vi "FPGA Close Reference.vi"(7 "Reset?":T1, 8 "error in (no error)":errorcluster, 11 "FPGA Session In":refnum<class "FPGA Interface Base.lvclass">) -> (0 "error out":errorcluster)   [LabVIEW 2010, in "FPGA Interface Base.lvclass"]
uses:
  <userlib>/_FPGA Interface Advanced Tools/FPGA Interface Base/FPGA Interface Base.lvclass
  <userlib>/_FPGA Interface Advanced Tools/FPGA Interface Wrapper/TypeDefs/Close Attribute.ctl
  <userlib>/_FPGA Interface Advanced Tools/FPGA Interface Base/FPGA Interface Base.lvclass/FPGA Interface Base.ctl
  <vilib>/Utility/error.llb/Error Cluster From Error Code.vi
  <userlib>/_FPGA Interface Advanced Tools/FPGA Interface Wrapper/FPGA Interface Wrapper.lvlib
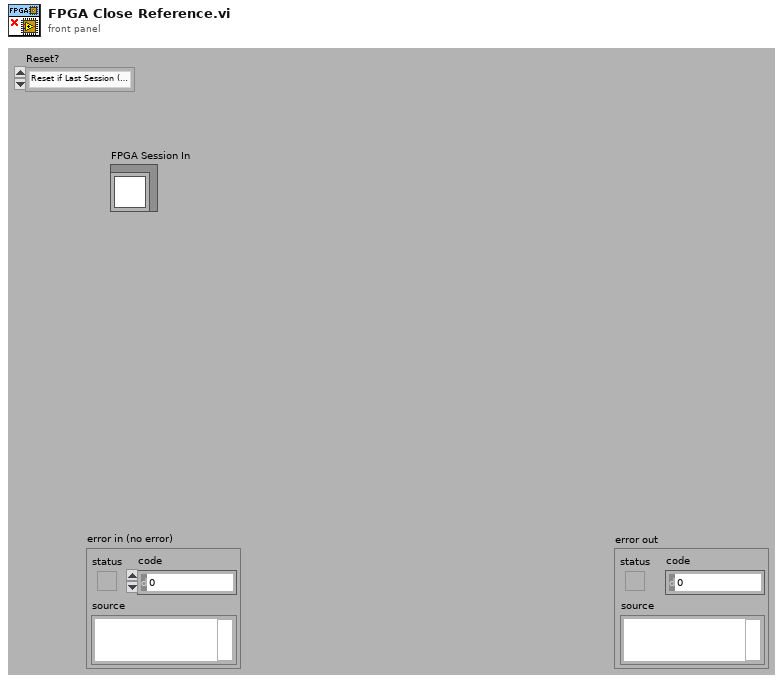
[diagram p1: front panel]
types:
  T1 = typedef "FPGA Interface Wrapper.lvlib/Close Attribute.ctl" = enum32{"Reset if Last Session (Default)", "No Reset"}
  T2 = typedef "FPGA Interface Base.lvclass/FPGA Session.ctl" = refnum<data-value>
  T3 = typedef "FPGA Interface Base.lvclass/FPGA Session Data.ctl" = cluster{"Session Out":u32, "Indicator Scalars":T4, "Indicator Arrays":T6, "Control Scalars":T4, "Control Arrays":T6, "TargetToHost FIFO Channels":T8, "HostToTarget FIFO Channels":T8, "All FIFOs":T9[], "IRQ Context Queue":refnum<queue>}
  T4 = typedef "FPGA Bitfile Utility.lvlib/Scalar Register Set.ctl" = cluster{"Boolean":T5[], "I8":T5[], "I16":T5[], "I32":T5[], "I64":T5[], "U8":T5[], "U16":T5[], "U32":T5[], "U64":T5[]}
  T5 = typedef "FPGA Bitfile Utility.lvlib/Scalar Register.ctl" = cluster{"Address":u32, "Name":string}
  T6 = typedef "FPGA Bitfile Utility.lvlib/Array Register Set.ctl" = cluster{"Boolean":T7[], "I8":T7[], "I16":T7[], "I32":T7[], "I64":T7[], "U8":T7[], "U16":T7[], "U32":T7[], "U64":T7[]}
  T7 = typedef "FPGA Bitfile Utility.lvlib/Array Register.ctl" = cluster{"Address":u32, "Num Elements":u32, "Name":string}
  T8 = typedef "FPGA Bitfile Utility.lvlib/FIFO Channel Set.ctl" = cluster{"Boolean":T9[], "I8":T9[], "I16":T9[], "I32":T9[], "I64":T9[], "U8":T9[], "U16":T9[], "U32":T9[], "U64":T9[]}
  T9 = typedef "FPGA Bitfile Utility.lvlib/FIFO Channel.ctl" = cluster{"Physical Channel":u32, "Name":string}
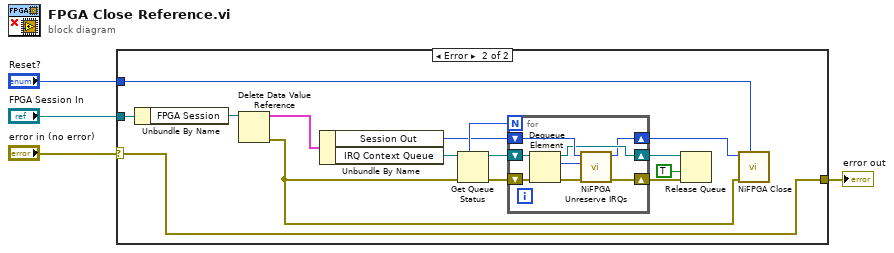
[diagram p0: block diagram]
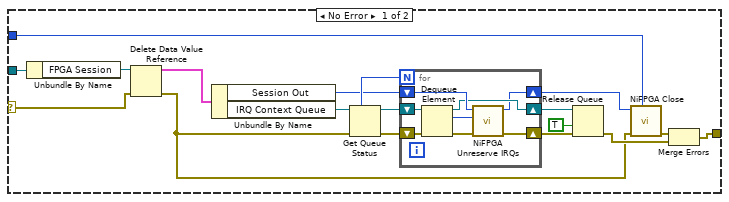
[diagram p2: hidden frame]
diagram:
  n1 = case shown="Error" "error in (no error)" {
    selector: "error in (no error)" -> [w12 w31]
    tunnel: [w7 w31] -> w3
    tunnel: "FPGA Session In" -> [w14 w37]
    tunnel: "Reset?" -> [w15 w38]
    frame No Error {
      n2 = Unbundle By Name(w14) -> ("FPGA Session"=w13:T2)
      n3 = Delete Data Value Reference(data value reference=w13, error in=w12) -> (data value=w11:T3, error out=w5:errorcluster)
      n4 = Unbundle By Name(w11) -> ("Session Out"=w10:u32, "IRQ Context Queue"=w9:refnum<queue>)
      n5 = Get Queue Status(queue=w9, error in (no error)=w5) -> (queue out=w22:refnum<queue>, max queue size=w20:i32, error out=w21:errorcluster)  [unwired: 1 in, 5 out]
      n6 = for {
        N: w20 -> [_]
        shift-right: [w26] -> w18
        shift-left: w21 -> [w29]
        shift-right: [w24] -> w19
        shift-left: w22 -> [w30]
        shift-right: [w23] -> w16
        shift-left: w10 -> [w25]
        n7 = Dequeue Element(queue=w30, error in (no error)=w29) -> (queue out=w24:refnum<queue>, element=w28:u32, error out=w27:errorcluster)  [unwired: 1 in, 1 out]
        n8 = call <userlib>:"NiFPGA Unreserve IRQs.vi"("error in (no error)"=w27, "Context"=w28, "Session In"=w25) -> ("error out"=w26:errorcluster, "Session Out"=w23:u32)  [unwired: 7 in]
      }
      n9 = Release Queue(queue=w19, force destroy? (F)=TRUE, error in (no error)=w18) -> (error out=w6:errorcluster)  [unwired: 2 out]
      n10 = call <userlib>:"NiFPGA Close.vi"("Attribute"=w15, "error in (no error)"=w5, "Session"=w16) -> ("error out"=w8:errorcluster)  [unwired: 7 in, 1 out]
      n11 = Merge Errors(w8, w6) -> (w7:errorcluster)
    }
    frame Error {
      n12 = Unbundle By Name(w37) -> ("FPGA Session"=w36:T2)
      n13 = Delete Data Value Reference(data value reference=w36) -> (data value=w35:T3, error out=w32:errorcluster)  [unwired: 1 in]
      n14 = Unbundle By Name(w35) -> ("Session Out"=w34:u32, "IRQ Context Queue"=w33:refnum<queue>)
      n15 = Get Queue Status(queue=w33, error in (no error)=w32) -> (queue out=w45:refnum<queue>, max queue size=w43:i32, error out=w44:errorcluster)  [unwired: 1 in, 5 out]
      n16 = for {
        N: w43 -> [_]
        shift-right: [w49] -> w41
        shift-left: w44 -> [w52]
        shift-right: [w47] -> w42
        shift-left: w45 -> [w53]
        shift-right: [w46] -> w39
        shift-left: w34 -> [w48]
        n17 = Dequeue Element(queue=w53, error in (no error)=w52) -> (queue out=w47:refnum<queue>, element=w51:u32, error out=w50:errorcluster)  [unwired: 1 in, 1 out]
        n18 = call <userlib>:"NiFPGA Unreserve IRQs.vi"("error in (no error)"=w50, "Context"=w51, "Session In"=w48) -> ("error out"=w49:errorcluster, "Session Out"=w46:u32)  [unwired: 7 in]
      }
      n19 = Release Queue(queue=w42, force destroy? (F)=TRUE, error in (no error)=w41) -> ()  [unwired: 3 out]
      n20 = call <userlib>:"NiFPGA Close.vi"("Attribute"=w38, "error in (no error)"=w32, "Session"=w39) -> ()  [unwired: 7 in, 2 out]
    }
  }
  "error out" <- w3
